vi "chart series set trendline equation.vi"(8 "error in (no error)":errorcluster, 11 "series":u32) -> (0 "error out":errorcluster, 3 "function return":u32(ring))   [LabVIEW 2015, in "xlsxwriter.lvlib"]
doc: "lxw_error chart_series_set_trendline_equation(lxw_chart_series series);"
uses:
  xlsxwriter.lvlib
  xlsxwriter.dll
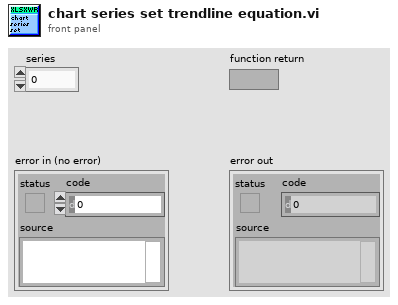
[diagram p1: front panel]
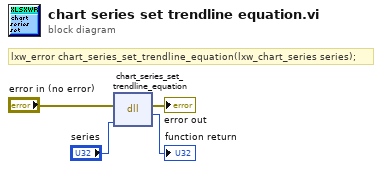
[diagram p0: block diagram]
diagram:
  # "lxw_error chart_series_set_trendline_equation(lxw_chart_series series);"
  n1 = dll-call lib="C:/Users/WDAGUtilityAccount/Desktop/lv_vis_added_cell/xlsxwriter.*" fn="chart_series_set_trendline_equation"(error in="error in (no error)", "series"="series") -> (error out=→"error out":errorcluster, →"function return":u32)  [unwired: 3 in, 1 out]
